vi "SetAngleHeading.vi"(2 "Desired Heading (rad)":dbl, 3 "Current Heading (rad)":dbl) -> (0 "Relative Angle Out (rad)":dbl, 1 "Relative Angle Out (deg)":dbl)   [LabVIEW 2011]
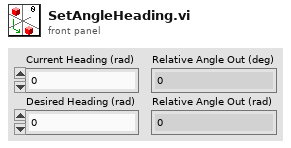
[diagram p1: front panel]
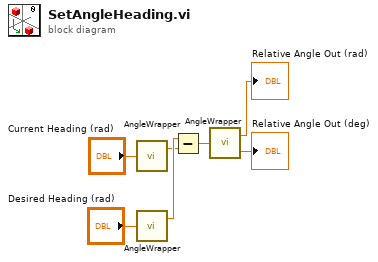
[diagram p0: block diagram]
diagram:
  n1 = call "AngleWrapper.vi"("Heading In (rad)"="Current Heading (rad)") -> ("Heading Out (rad)"=w4:dbl)  [unwired: 1 out]
  n2 = call "AngleWrapper.vi"("Heading In (rad)"="Desired Heading (rad)") -> ("Heading Out (rad)"=w5:dbl)  [unwired: 1 out]
  n3 = Subtract(x=w5, y=w4) -> (x-y=w3:dbl)
  n4 = call "AngleWrapper.vi"("Heading In (rad)"=w3) -> ("Heading Out (rad)"=→"Relative Angle Out (rad)":dbl, "Heading Out (deg)"=→"Relative Angle Out (deg)":dbl)
